vi "Find Engine Simulation Toolkit Custom Device.vi"(8 "error in (no error)":errorcluster, 10 "Name":string, 11 "Target in":refnum<k24>) -> (0 "error out":errorcluster, 2 "EST Custom Device":refnum<k24>, 3 "Target out":refnum<k24>)   [LabVIEW 2015, in "Engine Simulation Toolkit SysDef API.lvlib"]
uses:
  Engine Simulation Toolkit SysDef API.lvlib
  NationalInstruments.VeriStand.SystemDefinitionAPI
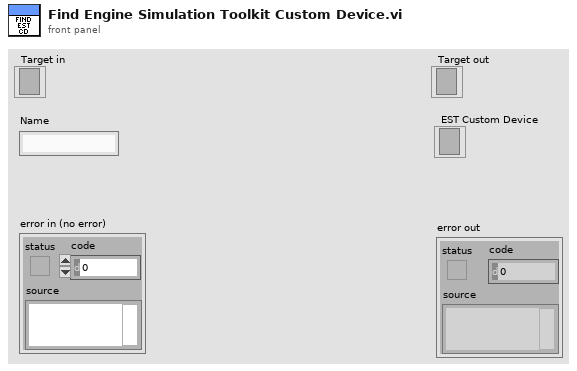
[diagram p1: front panel]
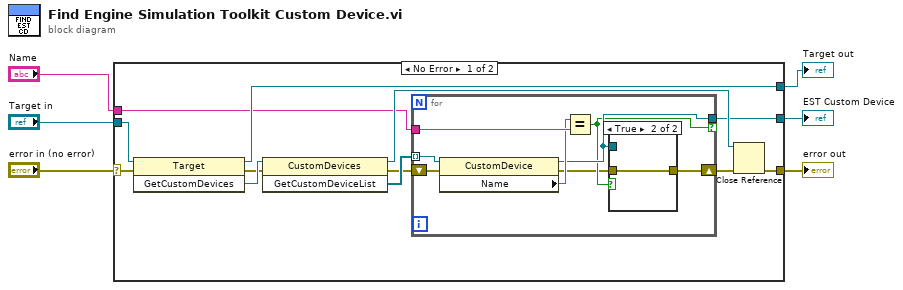
[diagram p0: block diagram]
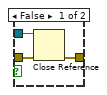
[diagram p2: hidden frame]
diagram:
  n1 = case shown="No Error" "error in (no error)" {
    selector: "error in (no error)" -> [w17 w32]
    tunnel: [w13 w32] -> w6
    tunnel: "Target in" -> [w18 w31]
    tunnel: [w14 w31] -> w3
    tunnel: "Name" -> [w10 _]
    tunnel: [w9 _] -> w1
    frame No Error {
      n2 = invoke class="Target" method="GetCustomDevices"(reference=w18, error in=w17) -> (reference out=w14:refnum<k24>, error out=w15:errorcluster, "GetCustomDevices"=w16:refnum<k24>)  [unwired: 1 in]
      n3 = invoke class="CustomDevices" method="GetCustomDeviceList"(reference=w16, error in=w15) -> (reference out=w12:refnum<k24>, error out=w7:errorcluster, "GetCustomDeviceList"=w11:refnum<k24>[])  [unwired: 1 in]
      n4 = for {
        tunnel: w11 -> [w26] mode=indexing
        tunnel: w10 -> [w25]
        tunnel: [w22] -> w9 if=w21
        shift-right: [w23] -> w8
        shift-left: w7 -> [w19]
        n5 = property class="CustomDevice"(reference=w26, error in=w19) -> (reference out=w22:refnum<k24>, error out=w20:errorcluster, "Name"=w24:string)
        n6 = Equal?(x=w24, y=w25) -> (x = y?=w21:bool)
        n7 = case shown="True" w21 {
          tunnel: w20 -> [w29 w30]
          tunnel: [w28 w30] -> w23
          tunnel: w22 -> [w27 _]
          frame False {
            n8 = Close Reference(reference=w27, error in (no error)=w29) -> (error out=w28:errorcluster)
          }
          frame True {
          }
        }
      }
      n9 = Close Reference(reference=w12, error in (no error)=w8) -> (error out=w13:errorcluster)
    }
    frame Error {
    }
  }
  "error out" <- w6
  "Target out" <- w3
  "EST Custom Device" <- w1
